vi "Write Save Images cont.vi"(8 "error in (no error)":errorcluster, 10 "Save Images cont":bool, 11 "HIJ Vision Camera App in":refnum<class "HIJ Vision Camera App.lvclass">) -> (0 "error out":errorcluster, 3 "HIJ Vision Camera App out":refnum<class "HIJ Vision Camera App.lvclass">)   [LabVIEW 2014, in "HIJ Vision Camera App.lvlib" / "HIJ Vision Camera App.lvclass"]
uses:
  HIJ Vision Camera App.lvclass
  HIJ Vision Camera App.lvclass/HIJ Vision Camera App.ctl
  HIJ Vision Application/HIJ Vision Application/HIJ Vision Application.lvclass/HIJ Vision Application.ctl
  <vilib>/ActorFramework/Message Enqueuer/Message Enqueuer.lvclass/Message Enqueuer.ctl
  HIJ Vision Application/HIJ Vision Application/Read Display Enq.vi
  <vilib>/ActorFramework/Message Enqueuer/Enqueue.vi
  <vilib>/ActorFramework/Message Priority Queue/Priority Enqueue.vi
  Display Actors/HIJ Vision Display/HIJ Vision Display Messages/Save Image Msg/Save Image Msg.lvclass
  <vilib>/ActorFramework/Message Enqueuer/Message Enqueuer.lvclass
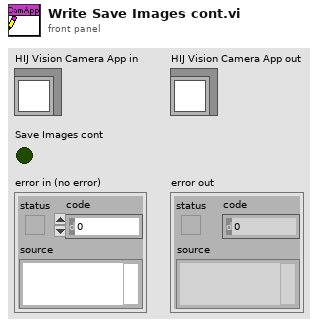
[diagram p1: front panel]
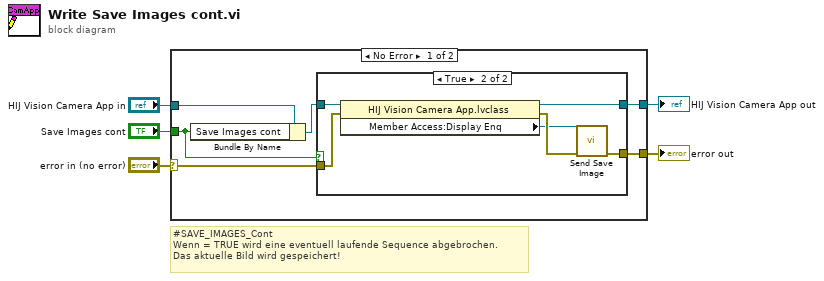
[diagram p0: block diagram]
diagram:
  # "#SAVE_IMAGES_Cont\nWenn = TRUE wird eine eventuell laufende Sequence abgebrochen.\nDas aktuelle Bild wird gespeichert!"
  n1 = case shown="No Error" "error in (no error)" {
    selector: "error in (no error)" -> [w6 w20]
    tunnel: [w11 w20] -> w4
    tunnel: [w9 w21] -> w2
    tunnel: "HIJ Vision Camera App in" -> [w7 w21]
    tunnel: "Save Images cont" -> [w10 _]
    frame No Error {
      n2 = Bundle By Name(cluster=w7, "Save Images cont"=w10) -> (w8:refnum<class "HIJ Vision Camera App.lvclass">)
      n3 = case shown="True" w10 {
        tunnel: [w12 w19] -> w11
        tunnel: [w13 w16] -> w9
        tunnel: w8 -> [w13 w18]
        tunnel: w6 -> [w12 w17]
        frame False {
        }
        frame True {
          n4 = property class="HIJ Vision Camera App.lvclass"(reference=w18, error in=w17) -> (reference out=w16:refnum<class "HIJ Vision Camera App.lvclass">, error out=w15:errorcluster, "Member Access:Display Enq"=w14:refnum<class "Message Enqueuer.lvclass">)
          n5 = call "Send Save Image.vi"("error in (no error)"=w15, "Message Enqueuer"=w14) -> ("error out"=w19:errorcluster)  [unwired: 8 in, 1 out]
        }
      }
    }
    frame Error {
    }
  }
  "error out" <- w4
  "HIJ Vision Camera App out" <- w2
